vi "BuildMenu.vi"(8 "error in (no error)":errorcluster, 10 "menu reference":refnum<k9>, 11 "Linear_Task in":refnum<class "Linear_Task.lvclass">) -> (0 "error out":errorcluster, 3 "Linear_Task out":refnum<class "Linear_Task.lvclass">)   [LabVIEW 2025, in "Linear_Task.lvlib" / "Linear_Task.lvclass"]
uses:
  Linear_Task.lvclass
  Linear_Task.lvclass/Linear_Task.ctl
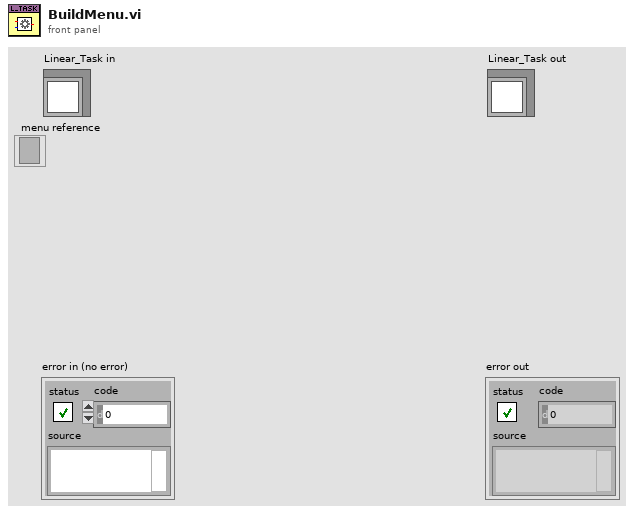
[diagram p1: front panel]
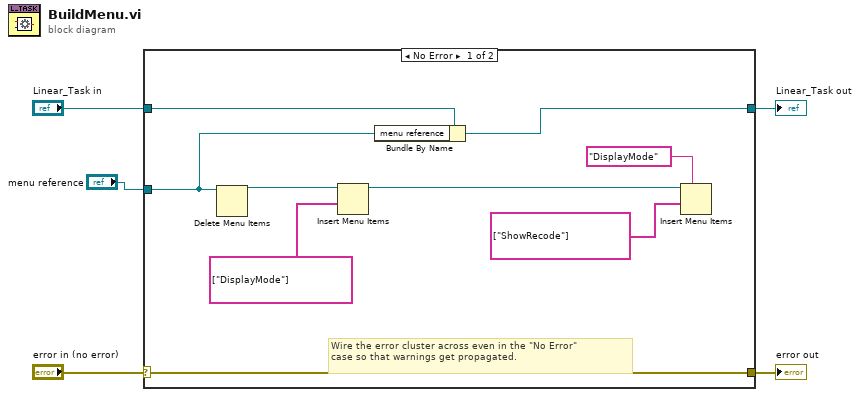
[diagram p0: block diagram]
diagram:
  n1 = case shown="No Error" "error in (no error)" {
    selector: "error in (no error)" -> [w14 w16]
    tunnel: [w14 w16] -> w4
    tunnel: [w7 w15] -> w2
    tunnel: "Linear_Task in" -> [w8 w15]
    tunnel: "menu reference" -> [w6 _]
    frame No Error {
      # "Wire the error cluster across even in the \"No Error\"\ncase so that warnings get propagated."
      n2 = Delete Menu Items(9:w6) -> (3:w12:refnum<k9>)  [unwired: 3 in, 1 out]
      n3 = Insert Menu Items(7:string[] ["DisplayMode"] ("item tags"), 9:w12) -> (3:w11:refnum<k9>)  [unwired: 4 in, 2 out]
      n4 = Bundle By Name(cluster=w8, "menu reference"=w6) -> (w7:refnum<class "Linear_Task.lvclass">)
      n5 = Insert Menu Items(5:"DisplayMode" ("menu tag"), 7:string[] ["ShowRecode"] ("item tags"), 9:w11) -> ()  [unwired: 3 in, 3 out]
    }
    frame Error {
    }
  }
  "error out" <- w4
  "Linear_Task out" <- w2
